vi "Recall.vi"(8 "error in (no error)":errorcluster, 9 "File Name ()":string, 10 "Data Type (0: Entire Instrument State)":u16(ring) items=["Entire Instrument State", "Segment Sweep Table", "Limit Table", "Power Sensor A", "Power Sensor B", "VBA Project", "Loss Compensation Table 1", "Loss Compensation Table 2", "Loss Compensation Table 3", "Loss Compensation Table 4", "Ripple Limit Table"], 11 "VISA resource name":refnum<visa-resource-name>) -> (0 "error out":errorcluster, 3 "VISA resource name out":refnum<visa-resource-name>)   [LabVIEW 2012, in "Tektronix TTR500 Series.lvlib"]
doc: "This VI recalls saved instrument data from a file."
uses:
  <instrlib>/Tektronix TTR500 Series/Tektronix TTR500 Series.lvlib
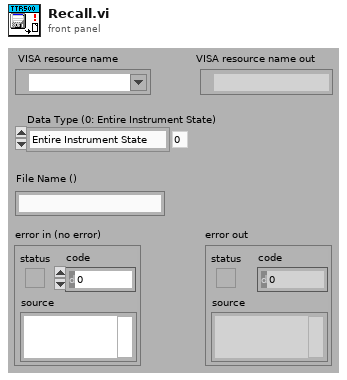
[diagram p1: front panel]
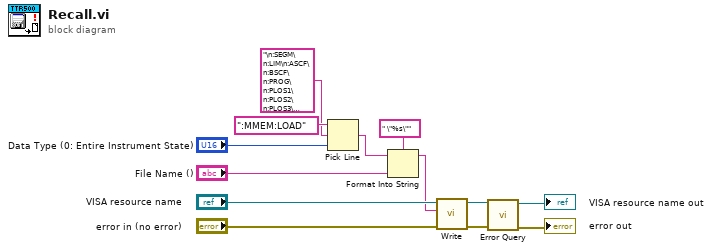
[diagram p0: block diagram]
diagram:
  n1 = Pick Line(string ("")=":MMEM:LOAD", multi-line string="\n:SEGM\n:LIM\n:ASCF\n:BSCF\n:PROG\n:PLOS1\n:PLOS2\n:PLOS3\n:PLOS4\n:RLIM", line index="Data Type (0: Entire Instrument State)") -> (output string=w7:string)
  n2 = Format Into String(format string=" \"%s\"", initial string=w7, "File Name ()") -> (resulting string=w10:string)  [unwired: 1 in, 1 out]
  n3 = call <instrlib>:"Write.vi"("error in (no error)"="error in (no error)", "String ()"=w10, "VISA resource name"="VISA resource name") -> ("error out"=w3:errorcluster, "VISA resource name out"=w4:refnum<visa-resource-name>)  [unwired: 6 in, 1 out]
  n4 = call <instrlib>:"Error Query.vi"("error in (no error)"=w3, "VISA resource name"=w4) -> ("error out"=→"error out":errorcluster, "VISA resource name out"=→"VISA resource name out":refnum<visa-resource-name>)  [unwired: 6 in, 2 out]
